vi "ex_Traffic_Lights_d.vi"() -> ()   [LabVIEW 2022 SP3]
uses:
  #typedef_Semaphore.ctl
  #typedef_Lights_States.ctl
  #typedef_Lights_ProgramData.ctl
  #typedef_Semaphores.ctl
  Timer/#typedef_TimerAction.ctl
panel:
  in  "stop":bool
  out "South":T1
  out "East":T1
  out "West":T1
  out "North":T1
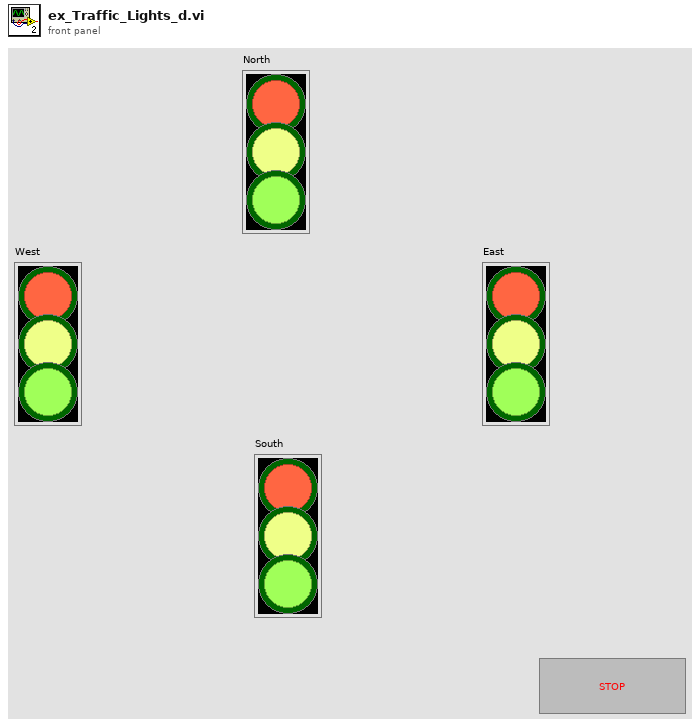
[diagram p1: front panel]
types:
  T1 = typedef "#typedef_Semaphore.ctl" = cluster{"Red":bool, "Yellow":bool, "Green":bool}
  T2 = typedef "#typedef_Lights_States.ctl" = enum16{"Initialize", "Idle", "NS_Green", "NS_Yellow", "NS_Red", "EW_Green", "EW_Yellow", "EW_Red", "ErrorHandler", "Exit"}
  T3 = typedef "#typedef_TimerAction.ctl" = enum16{"Reset", "TimeElapsed"}
  T4 = typedef "#typedef_Lights_ProgramData.ctl" = cluster{"Semaphores":T5, "NextTargetState":T2, "LightTimers":cluster{"NS_Green":dbl, "NS_Yellow":dbl, "NS_Red":dbl, "EW_Green":dbl, "EW_Yellow":dbl, "EW_Red":dbl}}
  T5 = typedef "#typedef_Semaphores.ctl" = cluster{"North":T1, "West":T1, "East":T1, "South":T1}
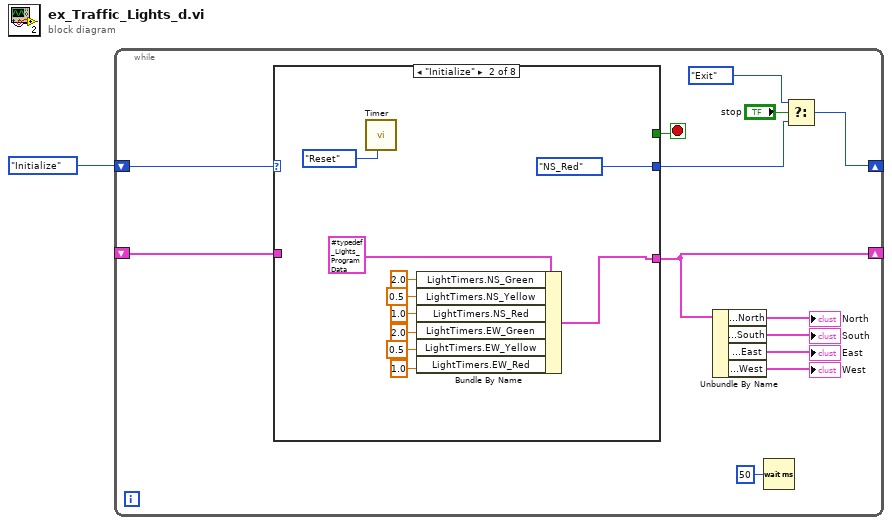
[diagram p0: block diagram]
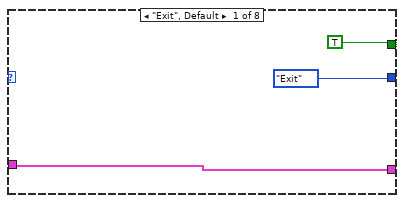
[diagram p2: hidden frame]
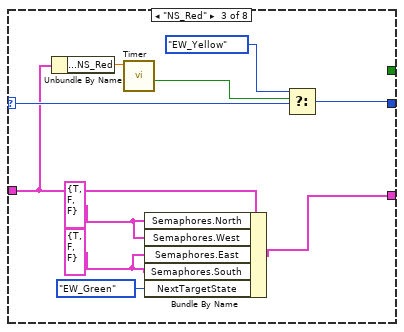
[diagram p3: hidden frame]
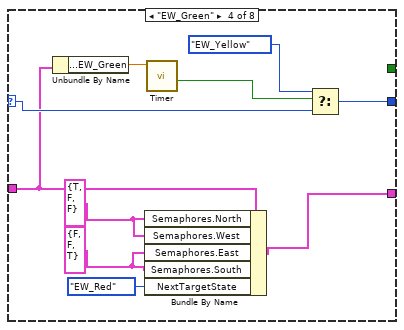
[diagram p4: hidden frame]
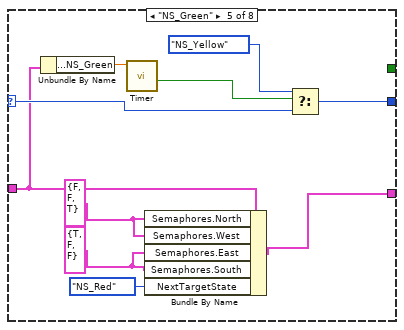
[diagram p5: hidden frame]
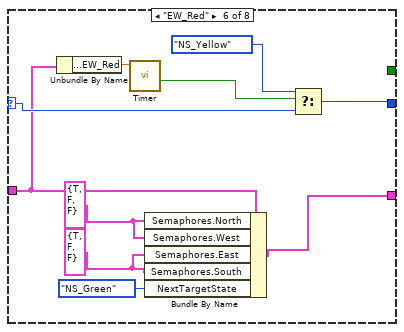
[diagram p6: hidden frame]
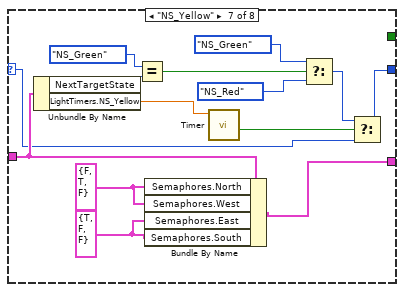
[diagram p7: hidden frame]
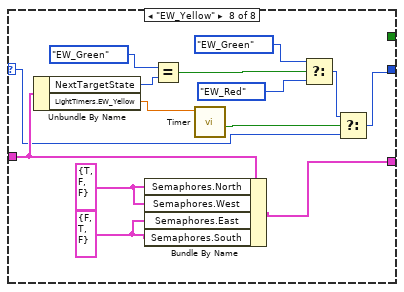
[diagram p8: hidden frame]
diagram:
  n1 = while {
    shift-right: [w3] -> _
    shift-left: #typedef_Lights_States."Initialize" ("Traffic_Light_States") -> [w14]
    shift-right: [w11] -> _
    shift-left: _ -> [w12]
    stop <- w13 stop-if-true
    n2 = case shown="\"Initialize\"" w14 {
      selector: w14 -> [_ _ w30 w39 w49 w59 w69 w82]
      tunnel: [#typedef_Lights_States."Exit" ("Traffic_Light_States") #typedef_Lights_States."NS_Red" ("Traffic_Light_States") w32 w40 w50 w60 w68 w83] -> w4
      tunnel: [w16 w24 w35 w45 w55 w65 w79 w93] -> w11
      tunnel: [TRUE _ _ _ _ _ _ _] -> w13
      tunnel: w12 -> [w16 _ w28 w38 w48 w58 w76 w90]
      frame "Exit", Default {
      }
      frame "Initialize" {
        n3 = call "Timer.vi"("Action (Time Elapsed)"=#typedef_TimerAction."Reset") -> ()  [unwired: 8 in, 3 out]
        n4 = Bundle By Name(cluster=T4 {"Semaphores"={"North"={"Red"=TRUE, "Yellow"=FALSE, "Green"=FALSE}, "West"={"Red"=TRUE, "Yellow"=FALSE, "Green"=FALSE}, "East"={"Red"=TRUE, "Yellow"=FALSE, "Green"=FALSE}, "South"={"Red"=TRUE, "Yellow"=FALSE, "Green"=FALSE}}, "NextTargetState"=enum."Initialize", "LightTimers"={"NS_Green"=0.0, "NS_Yellow"=0.0, "NS_Red"=0.0, "EW_Green"=0.0, "EW_Yellow"=0.0, "EW_Red"=0.0}} ("ProgramData"), "LightTimers.NS_Green"=2.0, "LightTimers.NS_Yellow"=0.5, "LightTimers.NS_Red"=1.0, "LightTimers.EW_Green"=2.0, "LightTimers.EW_Yellow"=0.5, "LightTimers.EW_Red"=1.0) -> (w24:T4)
      }
      frame "NS_Red" {
        w36 = T1 {"Red"=TRUE, "Yellow"=FALSE, "Green"=FALSE} ("Semaphores.North")
        w37 = T1 {"Red"=TRUE, "Yellow"=FALSE, "Green"=FALSE} ("Semaphores.North")
        n5 = Unbundle By Name(w28) -> ("LightTimers.NS_Red"=w29:dbl)
        n6 = call "Timer.vi"("Time To Elapse"=w29) -> ("Time Elapsed?"=w33:bool)  [unwired: 8 in, 2 out]
        n7 = Bundle By Name(cluster=w28, "Semaphores.North"=w37, "Semaphores.West"=w37, "Semaphores.East"=w36, "Semaphores.South"=w36, "NextTargetState"=#typedef_Lights_States."EW_Green" ("PreviousState")) -> (w35:T4)
        n8 = Select(t=#typedef_Lights_States."EW_Yellow" ("Traffic_Light_States"), s=w33, f=w30) -> (s? t:f=w32:T2)
      }
      frame "EW_Green" {
        w46 = T1 {"Red"=FALSE, "Yellow"=FALSE, "Green"=TRUE} ("Semaphores.North")
        w47 = T1 {"Red"=TRUE, "Yellow"=FALSE, "Green"=FALSE} ("Semaphores.North")
        n9 = Unbundle By Name(w38) -> ("LightTimers.EW_Green"=w43:dbl)
        n10 = Bundle By Name(cluster=w38, "Semaphores.North"=w47, "Semaphores.West"=w47, "Semaphores.East"=w46, "Semaphores.South"=w46, "NextTargetState"=#typedef_Lights_States."EW_Red" ("PreviousState")) -> (w45:T4)
        n11 = call "Timer.vi"("Time To Elapse"=w43) -> ("Time Elapsed?"=w41:bool)  [unwired: 8 in, 2 out]
        n12 = Select(t=#typedef_Lights_States."EW_Yellow" ("Traffic_Light_States"), s=w41, f=w39) -> (s? t:f=w40:T2)
      }
      frame "NS_Green" {
        w56 = T1 {"Red"=TRUE, "Yellow"=FALSE, "Green"=FALSE} ("Semaphores.North")
        w57 = T1 {"Red"=FALSE, "Yellow"=FALSE, "Green"=TRUE} ("Semaphores.North")
        n13 = Unbundle By Name(w48) -> ("LightTimers.NS_Green"=w51:dbl)
        n14 = call "Timer.vi"("Time To Elapse"=w51) -> ("Time Elapsed?"=w53:bool)  [unwired: 8 in, 2 out]
        n15 = Bundle By Name(cluster=w48, "Semaphores.North"=w57, "Semaphores.West"=w57, "Semaphores.East"=w56, "Semaphores.South"=w56, "NextTargetState"=#typedef_Lights_States."NS_Red" ("PreviousState")) -> (w55:T4)
        n16 = Select(t=#typedef_Lights_States."NS_Yellow" ("Traffic_Light_States"), s=w53, f=w49) -> (s? t:f=w50:T2)
      }
      frame "EW_Red" {
        w66 = T1 {"Red"=TRUE, "Yellow"=FALSE, "Green"=FALSE} ("Semaphores.North")
        w67 = T1 {"Red"=TRUE, "Yellow"=FALSE, "Green"=FALSE} ("Semaphores.North")
        n17 = Unbundle By Name(w58) -> ("LightTimers.EW_Red"=w61:dbl)
        n18 = call "Timer.vi"("Time To Elapse"=w61) -> ("Time Elapsed?"=w63:bool)  [unwired: 8 in, 2 out]
        n19 = Bundle By Name(cluster=w58, "Semaphores.North"=w67, "Semaphores.West"=w67, "Semaphores.East"=w66, "Semaphores.South"=w66, "NextTargetState"=#typedef_Lights_States."NS_Green" ("PreviousState")) -> (w65:T4)
        n20 = Select(t=#typedef_Lights_States."NS_Yellow" ("Traffic_Light_States"), s=w63, f=w59) -> (s? t:f=w60:T2)
      }
      frame "NS_Yellow" {
        w80 = T1 {"Red"=TRUE, "Yellow"=FALSE, "Green"=FALSE} ("Semaphores.North")
        w81 = T1 {"Red"=FALSE, "Yellow"=TRUE, "Green"=FALSE} ("Semaphores.North")
        n21 = Unbundle By Name(w76) -> ("NextTargetState"=w75:T2, "LightTimers.NS_Yellow"=w72:dbl)
        n22 = Equal?(x=#typedef_Lights_States."NS_Green" ("Traffic_Light_States"), y=w75) -> (x = y?=w73:bool)
        n23 = Bundle By Name(cluster=w76, "Semaphores.North"=w81, "Semaphores.West"=w81, "Semaphores.East"=w80, "Semaphores.South"=w80) -> (w79:T4)
        n24 = call "Timer.vi"("Time To Elapse"=w72) -> ("Time Elapsed?"=w71:bool)  [unwired: 8 in, 2 out]
        n25 = Select(t=#typedef_Lights_States."NS_Green" ("Traffic_Light_States"), s=w73, f=#typedef_Lights_States."NS_Red" ("Traffic_Light_States")) -> (s? t:f=w70:T2)
        n26 = Select(t=w70, s=w71, f=w69) -> (s? t:f=w68:T2)
      }
      frame "EW_Yellow" {
        w94 = T1 {"Red"=FALSE, "Yellow"=TRUE, "Green"=FALSE} ("Semaphores.North")
        w95 = T1 {"Red"=TRUE, "Yellow"=FALSE, "Green"=FALSE} ("Semaphores.North")
        n27 = Unbundle By Name(w90) -> ("NextTargetState"=w89:T2, "LightTimers.EW_Yellow"=w86:dbl)
        n28 = Bundle By Name(cluster=w90, "Semaphores.North"=w95, "Semaphores.West"=w95, "Semaphores.East"=w94, "Semaphores.South"=w94) -> (w93:T4)
        n29 = Equal?(x=#typedef_Lights_States."EW_Green" ("Traffic_Light_States"), y=w89) -> (x = y?=w87:bool)
        n30 = call "Timer.vi"("Time To Elapse"=w86) -> ("Time Elapsed?"=w85:bool)  [unwired: 8 in, 2 out]
        n31 = Select(t=#typedef_Lights_States."EW_Green" ("Traffic_Light_States"), s=w87, f=#typedef_Lights_States."EW_Red" ("Traffic_Light_States")) -> (s? t:f=w84:T2)
        n32 = Select(t=w84, s=w85, f=w82) -> (s? t:f=w83:T2)
      }
    }
    n33 = Unbundle By Name(w11) -> ("Semaphores.North"=→"North":T1, "Semaphores.South"=→"South":T1, "Semaphores.East"=→"East":T1, "Semaphores.West"=→"West":T1)
    n34 = Wait (ms)(milliseconds to wait=u32 50) -> ()  [unwired: 1 out]
    n35 = Select(t=#typedef_Lights_States."Exit" ("Traffic_Light_States"), s="stop", f=w4) -> (s? t:f=w3:T2)
  }
